vi "Get Server DLL Path.vi"() -> (0 "Server dll path":path)   [LabVIEW 2019, in "Data Marshal Server.lvlib" / "gprc-lvsupport.lvlib"]
uses:
  gprc-lvsupport.lvlib
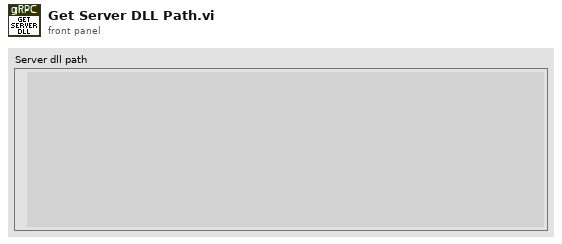
[diagram p1: front panel]
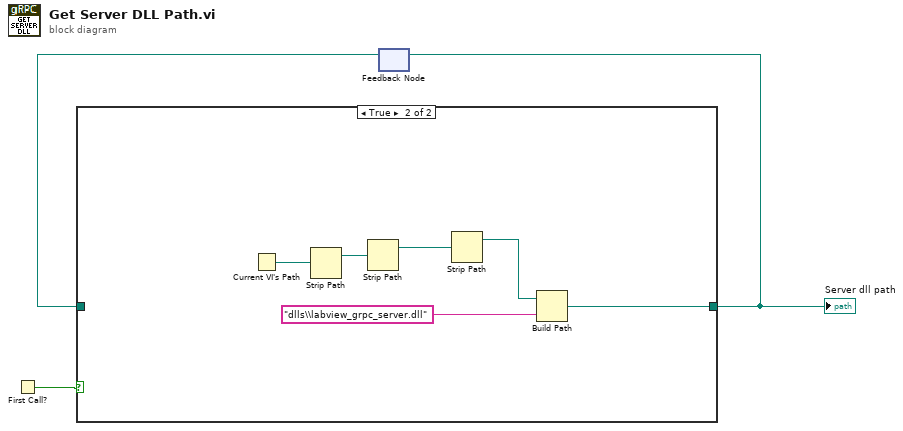
[diagram p0: block diagram]
diagram:
  n1 = First Call?() -> (First Call?: T/F=w3:bool)
  n2 = feedback #1() -> (w1:path)  [unwired: 1 in]
  n3 = case shown="True" w3 {
    tunnel: [w4 w7] -> w2
    tunnel: w1 -> [w4 _]
    frame False {
    }
    frame True {
      n4 = Current VI's Path() -> (path=w9:path)
      n5 = Strip Path(path=w9) -> (stripped path=w10:path)  [unwired: 1 out]
      n6 = Strip Path(path=w10) -> (stripped path=w6:path)  [unwired: 1 out]
      n7 = Strip Path(path=w6) -> (stripped path=w5:path)  [unwired: 1 out]
      n8 = Build Path(base path=w5, name or relative path="dlls\\labview_grpc_server.dll") -> (appended path=w7:path)
    }
  }
  "Server dll path" <- w2
  n9 = feedback-in #1(w2) -> ()
